vi "WristExecuteLogic.vi"(8 "error in (no error)":errorcluster, 11 "EncoderPos (deg)":dbl) -> (0 "error out":errorcluster, 3 "MotorDmd":dbl)   [LabVIEW 2023]
uses:
  <vilib>/Rock Robotics/WPI/ThirdParty/JAS_Junk/TrajLib/VI/BoolCmd_Recv_Internal.vi
  <vilib>/Rock Robotics/WPI/ThirdParty/JAS_Junk/TrajLib/Util_GetTime.vi
  <vilib>/Rock Robotics/WPI/ThirdParty/JAS_Junk/TrajLib/VI/MathUtil_RateOfChange.vi
  <vilib>/Rock Robotics/WPI/ThirdParty/JAS_Junk/TrajLib/VI/BoolCmd_ObtainQueue.vi
  <vilib>/Rock Robotics/WPI/ThirdParty/JAS_Junk/TrajLib/VI/Util_GetTime_U32.vi
  Elevator/ElevatorGlobal.vi
  WristGlobal.vi
  <vilib>/Rock Robotics/SystemInterfaces/Utilities/FPGA_UtilitiesRead LocalTime.vi
  <vilib>/Rock Robotics/WPI/ThirdParty/JAS_Junk/TrajLib/VI/Util_GetTime_U64.vi
  <vilib>/Rock Robotics/WPI/ThirdParty/JAS_Junk/TrajLib/Trajectory_Library.lvlib
  <vilib>/Rock Robotics/WPI/ThirdParty/JAS_Junk/TrajLib/Enum/DCMOTOR_TYPES_ENUM.ctl
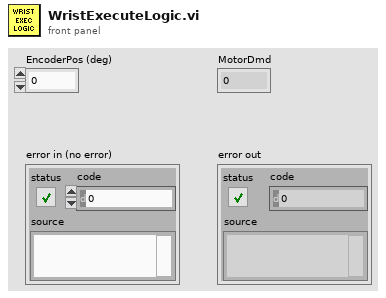
[diagram p1: front panel]
types:
  T1 = typedef "Trajectory_Library.lvlib/DCMOTOR_TYPES_ENUM.ctl" = enum16{"CIM", "AndyMark 9015", "Andy Mark RS 775 125", "Bag", "BaneBots RS 550", "BaneBots RS 775", "Falcon 500", "Mini CIM", "NEO", "NEO 550", "Romi BuiltIn", "Vex 775 Pro", "Snow Blower AM 2235A", "Bosch Seat AM 3493", "Falcon 500 FOC", "Kraken X60", "Kraken X60 FOC", "NEO Vortex"}
  T2 = typedef "Trajectory_Library.lvlib/LINEAR_SYSTEM_ID_SINGLE_JOINT_ARM_MODEL.ctl" = cluster{"DCMOTOR_TYPES":T1, "Num Motors":i32, "ArmLength_M":dbl, "massKg":dbl, "Gearing":dbl, "MOI kgm2":dbl, "Estimate MOI":bool}
  T3 = typedef "Trajectory_Library.lvlib/LINEAR_SYSTEM_LOOP_SNGJNTARM_CTRL_PARAMS.ctl" = cluster{"Ang Model Std Dev Rad":dbl, "Ang Meas Std Dev Rad":dbl, "Ang Ctrl Tol Rad":dbl, "Max Ctrl Out V":dbl, "Vel Model Std Dev Rad/Sec":dbl, "Vel Ctrl Tol Rad/Sec":dbl}
  T4 = typedef "Trajectory_Library.lvlib/PosCtrl_Tuning_Type.ctl" = cluster{"Slope":dbl, "Offset":dbl, "Error Deadband":dbl, "At Reference Count":i32, "Negate Output":bool, "Max Allowd Position":dbl, "Min Allowd Position":dbl, "Kd":dbl, "FilterDerivative":bool}
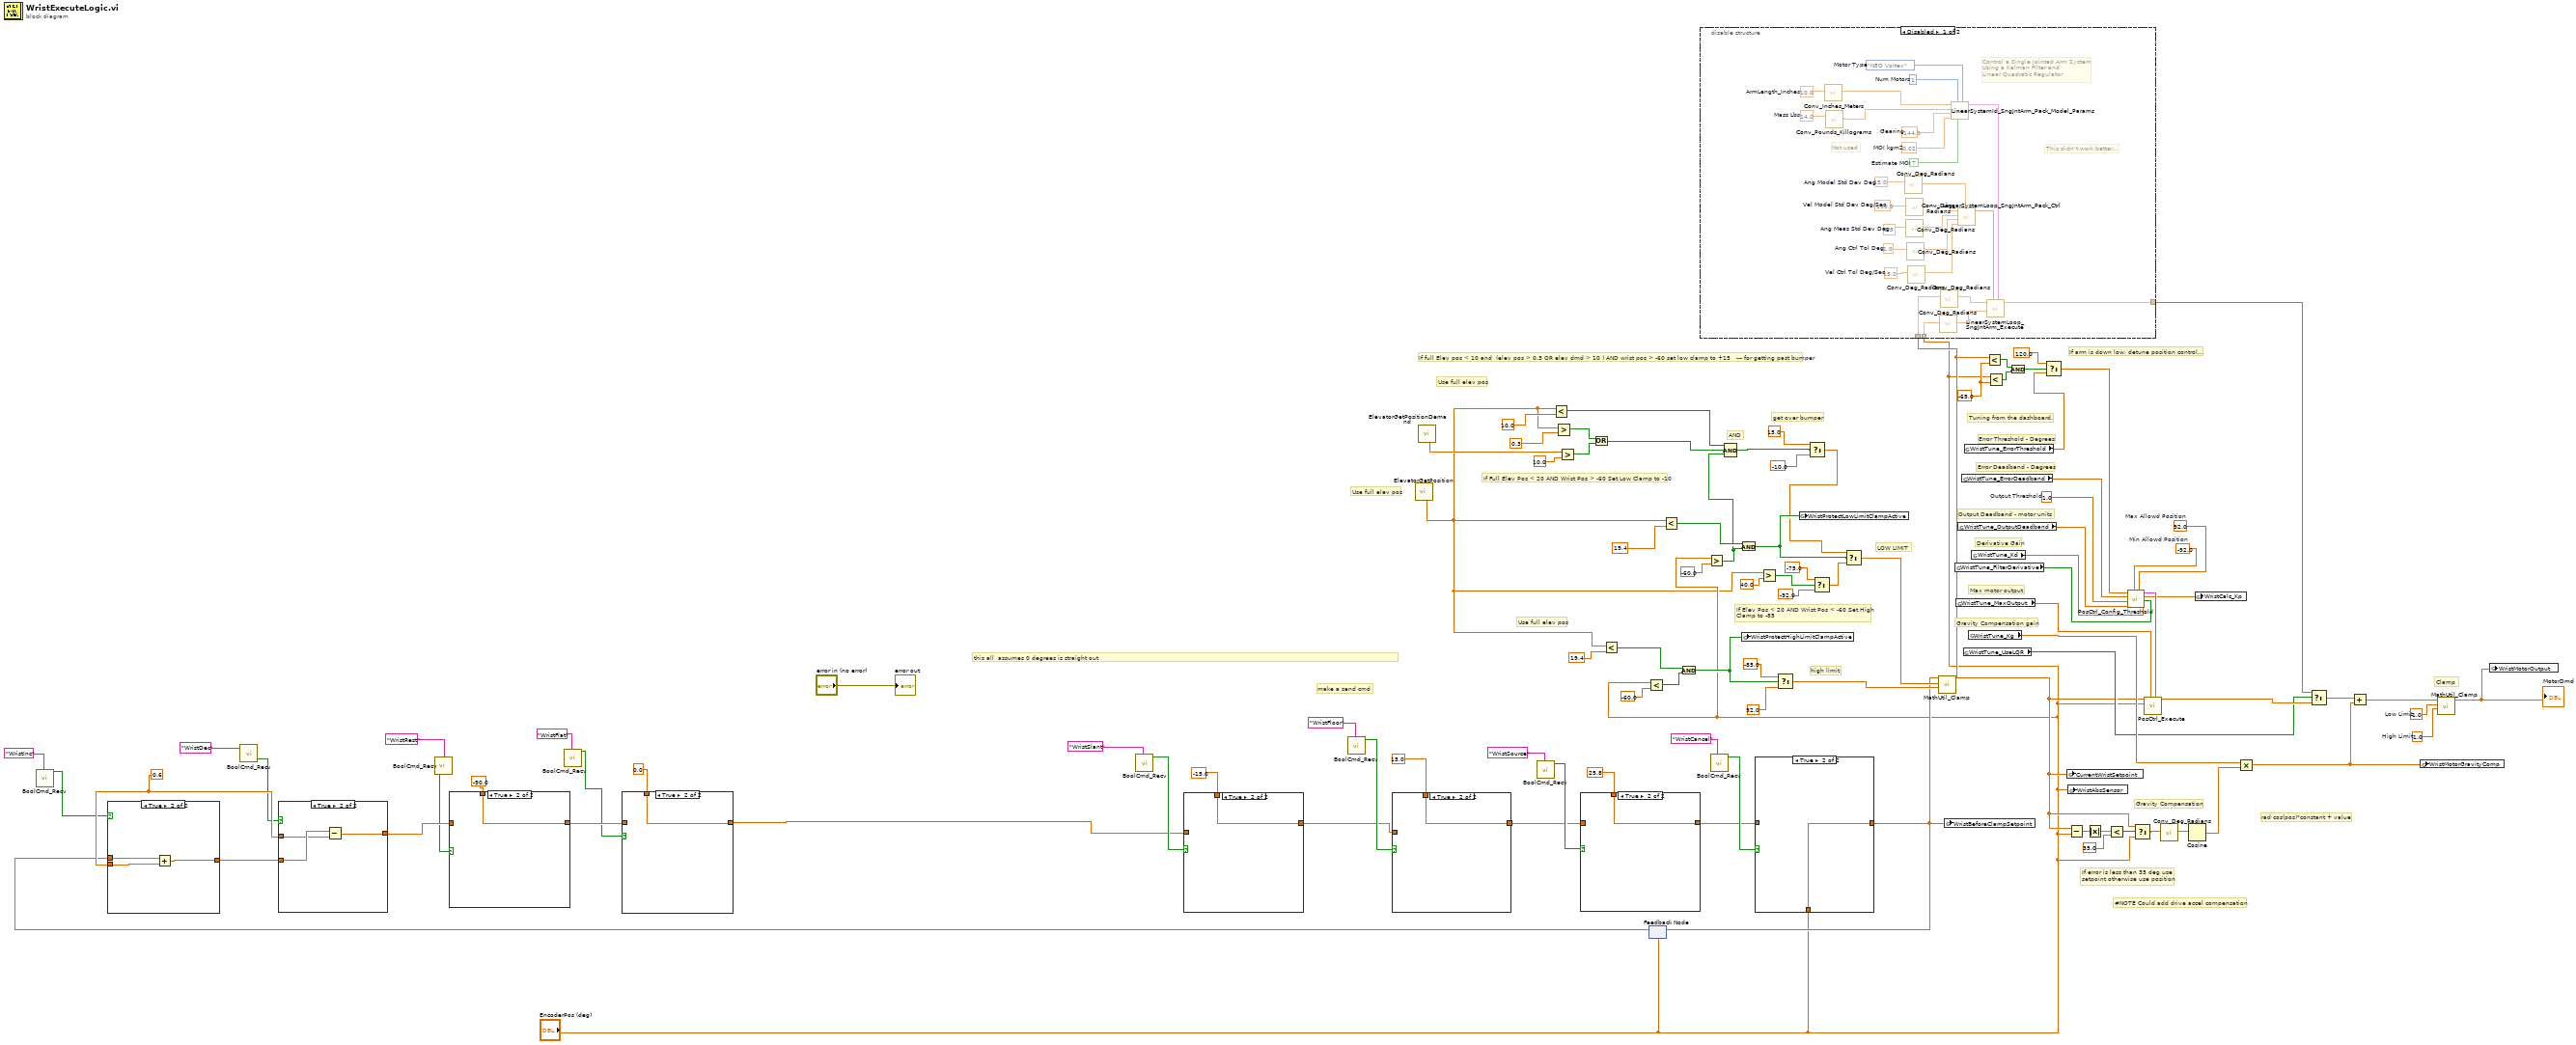
[diagram p0: block diagram]
diagram:
  w26 = -92.0  # Min Allowd Position
  w27 = 92.0  # Max Allowd Position
  w36 = -65.0 ("y")
  w99 = 1.0  # Output Threshold
  w97 = 1.0  # High Limit
  w98 = -1.0  # Low Limit
  w93 = 0.6 ("x")
  # "make a send cmd"
  # "LOW LIMIT"
  # "get over bumper"
  # "AND"
  # "Use full elev pos"
  # "If full Elev pos < 10 and  (elev pos > 0.3 OR elev dmd > 10 ) AND wrist pos > -60 set low clamp to +15   --- for getting past bumper"
  # "#NOTE Could add drive accel compensation"
  # "Use full elev pos"
  # "Use full elev pos"
  # "If arm is down low, detune position control..."
  # "If error is less than 35 deg use\nsetpoint otherwise use position"
  # "Gravity Compensation gain"
  # "Tuning from the dashboard."
  # "Max motor output"
  # "Derivative Gain"
  # "Output Deadband - motor units"
  # "Error Deadband - Degrees"
  # "Error Threshold - Degrees"
  # "If Elev Pos < 20 AND Wrist Pos < -60 Set High\nClamp to -85"
  # "If Full Elev Pos < 20 AND Wrist Pos > -60 Set Low Clamp to -10"
  # "high limit"
  # "Gravity Compensation"
  # "rad cos(pos)*constant + value"
  # "Clamp"
  # "this all  assumes 0 degrees is straight out"
  n1 = call <vilib>:"BoolCmd_Recv.vi"("Command Name"="WristInc") -> ("New Request"=w82:bool)  [unwired: 9 in, 1 out]
  n2 = call <vilib>:"BoolCmd_Recv.vi"("Command Name"="WristDec") -> ("New Request"=w84:bool)  [unwired: 9 in, 1 out]
  n3 = call <vilib>:"BoolCmd_Recv.vi"("Command Name"="WristRest") -> ("New Request"=w80:bool)  [unwired: 9 in, 1 out]
  n4 = call <vilib>:"BoolCmd_Recv.vi"("Command Name"="WristFlat") -> ("New Request"=w86:bool)  [unwired: 9 in, 1 out]
  n5 = call <vilib>:"BoolCmd_Recv.vi"("Command Name"="WristSlant") -> ("New Request"=w88:bool)  [unwired: 9 in, 1 out]
  n6 = call <vilib>:"BoolCmd_Recv.vi"("Command Name"="WristFloor") -> ("New Request"=w5:bool)  [unwired: 9 in, 1 out]
  n7 = call "ElevatorGetPosition.vi"() -> ("ElevFullHeight"=w10:dbl)  [unwired: 9 in, 2 out]
  n8 = call "ElevatorGetPositionDemand.vi"() -> ("ElevatorFullDmdInches"=w17:dbl)  [unwired: 8 in, 2 out]
  n9 = call <vilib>:"BoolCmd_Recv.vi"("Command Name"="WristSource") -> ("New Request"=w59:bool)  [unwired: 9 in, 1 out]
  n10 = Less?(x=w10, y=10.0) -> (x < y?=w23:bool)
  n11 = Greater?(x=w10, y=0.3) -> (0:w15:bool)
  n12 = Greater?(x=w17, y=10.0) -> (0:w14:bool)
  n13 = Or(x=w15, y=w14) -> (x .or. y?=w13:bool)
  n14 = Less?(x=w10, y=19.4) -> (x < y?=w67:bool)
  n15 = Less?(x="EncoderPos (deg)", y=-60.0) -> (x < y?=w65:bool)
  n16 = feedback #1("EncoderPos (deg)") -> (w89:dbl)
  n17 = case shown="True" w82 {
    tunnel: w89 -> [w101 w103]
    tunnel: [w101 w104] -> w90
    tunnel: w93 -> [_ w102]
    frame False {
    }
    frame True {
      n18 = Add(x=w103, y=w102) -> (x+y=w104:dbl)
    }
  }
  n19 = case shown="True" w84 {
    tunnel: w90 -> [w105 w107]
    tunnel: [w105 w108] -> w91
    tunnel: w93 -> [_ w106]
    frame False {
    }
    frame True {
      n20 = Subtract(x=w107, y=w106) -> (x-y=w108:dbl)
    }
  }
  n21 = case shown="True" w80 {
    tunnel: w91 -> [w109 _]
    tunnel: [w109 w110] -> w92
    tunnel: -90.0 ("Numeric") -> [_ w110]
    frame False {
    }
    frame True {
    }
  }
  n22 = case shown="True" w86 {
    tunnel: w92 -> [w111 _]
    tunnel: [w111 w112] -> w1
    tunnel: 0.0 ("Result") -> [_ w112]
    frame False {
    }
    frame True {
    }
  }
  n23 = case shown="True" w88 {
    tunnel: w1 -> [w113 _]
    tunnel: [w113 w114] -> w4
    tunnel: -15.0 ("Result") -> [_ w114]
    frame False {
    }
    frame True {
    }
  }
  n24 = case shown="True" w5 {
    tunnel: w4 -> [w115 _]
    tunnel: [w115 w116] -> w3
    tunnel: 15.0 ("Result") -> [_ w116]
    frame False {
    }
    frame True {
    }
  }
  n25 = case shown="True" w59 {
    tunnel: [w117 w118] -> w57
    tunnel: 25.8 ("Result") -> [_ w118]
    tunnel: w3 -> [w117 _]
    frame False {
    }
    frame True {
    }
  }
  n26 = Less?(x=w10, y=19.4) -> (x < y?=w63:bool)
  n27 = And(x=w67, y=w65) -> (x .and. y?=w54:bool)
  n28 = Greater?(x="EncoderPos (deg)", y=-60.0) -> (0:w22:bool)
  n29 = call <vilib>:"BoolCmd_Recv.vi"("Command Name"="WristCancel") -> ("New Request"=w77:bool)  [unwired: 9 in, 1 out]
  n30 = Compound Arithmetic op=AND(w23, w13, w22) -> (w19:bool)
  n31 = And(x=w63, y=w22) -> (x .and. y?=w55:bool)
  n32 = global write "WristGlobal.vi" "WristProtectHighLimitClampActive"(w54) -> ()
  n33 = case shown="True" w77 {
    tunnel: w57 -> [w119 _]
    tunnel: [w119 w120] -> w56
    tunnel: "EncoderPos (deg)" -> [_ w120]
    frame False {
    }
    frame True {
    }
  }
  n34 = feedback-in #1(w56) -> ()
  n35 = Greater?(x=w10, y=40.0) -> (0:w8:bool)
  n36 = Select(t=-85.0, s=w54, f=92.0) -> (s? t:f=w68:dbl)
  n37 = global write "WristGlobal.vi" "WristProtectLowLimitClampActive"(w55) -> ()
  n38 = Select(t=15.0, s=w19, f=-10.0 ("t")) -> (s? t:f=w18:dbl)
  n39 = Select(t=-75.0, s=w8, f=-92.0) -> (s? t:f=w11:dbl)
  n40 = Select(t=w18, s=w55, f=w11) -> (s? t:f=w61:dbl)
  n41 = call <vilib>:"MathUtil_Clamp.vi"("High Limit"=w68, "Low Limit"=w61, "Value"=w56) -> ("Result"=w33:dbl)  [unwired: 8 in]
  n42 = disable-structure shown="Disabled" {
    disable-tunnel: [w123 _] -> w38
    disable-tunnel: w33 -> [w122 _]
    disable-tunnel: "EncoderPos (deg)" -> [w121 _]
    frame Disabled {
      w130 = 100.0  # Vel Model Std Dev Deg/Sec
      w129 = 0.5  # Ang Meas Std Dev Deg
      w128 = 1.0  # Ang Ctrl Tol Deg
      w127 = 15.0  # Vel Ctrl Tol Deg/Sec
      w132 = 25.0  # Ang Model Std Dev Deg
      w142 = TRUE  # Estimate MOI
      w143 = 0.02  # MOI kgm2
      w137 = 10.0  # ArmLength_Inches
      w144 = 144.0  # Gearing
      w135 = 14.0  # Mass Lbs
      w145 = 1  # Num Motors
      w146 = DCMOTOR_TYPES_ENUM."NEO Vortex"  # Motor Type
      # "This didn't work better..."
      # "Not used"
      # "Control a Single Jointed Arm System\nUsing a Kalman Filter and \nLinear Quadratic Regulator"
      n43 = call <vilib>:"Conv_Inches_Meters.vi"("INCH"=w137) -> ("Meters"=w136:dbl)  [unwired: 10 in]
      n44 = call <vilib>:"Conv_Pounds_Killograms.vi"("Pounds"=w135) -> ("Killograms"=w134:dbl)  [unwired: 10 in]
      n45 = call <vilib>:"Conv_Deg_Radians.vi"("Degress"=w132) -> ("Radians"=w133:dbl)  [unwired: 10 in]
      n46 = call <vilib>:"Conv_Deg_Radians.vi"("Degress"=w129) -> ("Radians"=w126:dbl)  [unwired: 10 in]
      n47 = call <vilib>:"Conv_Deg_Radians.vi"("Degress"=w130) -> ("Radians"=w131:dbl)  [unwired: 10 in]
      n48 = call <vilib>:"Conv_Deg_Radians.vi"("Degress"=w128) -> ("Radians"=w125:dbl)  [unwired: 10 in]
      n49 = call <vilib>:"Conv_Deg_Radians.vi"("Degress"=w127) -> ("Radians"=w124:dbl)  [unwired: 10 in]
      n50 = call <vilib>:"Conv_Deg_Radians.vi"("Degress"=w121) -> ("Radians"=w139:dbl)  [unwired: 10 in]
      n51 = call <vilib>:"Conv_Deg_Radians.vi"("Degress"=w122) -> ("Radians"=w138:dbl)  [unwired: 10 in]
      n52 = call <vilib>:"LinearSystemId_SngJntArm_Pack_Model_Params.vi"("DCMOTOR_TYPES"=w146, "Estimate MOI"=w142, "Num Motors"=w145, "MOI kgm2"=w143, "Gearing"=w144, "massKg"=w134, "ArmLength_M"=w136) -> ("SngJntArmSim_Model _Params"=w141:T2)  [unwired: 4 in]
      n53 = call <vilib>:"LinearSystemLoop_SngJntArm_Pack_Ctrl.vi"("Ang Model Std Dev Rad"=w133, "Vel Ctrl Tol Rad/Sec"=w124, "Ang Ctrl Tol Rad"=w125, "Ang Meas Std Dev Rad"=w126, "Vel Model Std Dev Rad/Sec"=w131) -> ("LinearSystemLoop_SngJntArm_Ctrl_Params"=w140:T3)  [unwired: 6 in]
      n54 = call <vilib>:"LinearSystemLoop_SngJntArm_Execute.vi"("LinearSystem_ID_SngJntArm_Model"=w141, "LinearSystem_SngJntArm_Ctrl_Params"=w140, "Process Variable\nRadians"=w139, "Ang Pos SP Rad"=w138) -> ("Motor Dmd"=w123:dbl)  [unwired: 3 in, 4 out]
    }
    frame Enabled {
    }
  }
  n55 = global write "WristGlobal.vi" "WristBeforeClampSetpoint"(w56) -> ()
  n56 = global read "WristGlobal.vi" "WristTune_FilterDerivative"() -> (w48:bool)
  n57 = global read "WristGlobal.vi" "WristTune_MaxOutput"() -> (w50:dbl)
  n58 = global read "WristGlobal.vi" "WristTune_OutputDeadband"() -> (w52:dbl)
  n59 = global read "WristGlobal.vi" "WristTune_ErrorDeadband"() -> (w53:dbl)
  n60 = global read "WristGlobal.vi" "WristTune_UseLQR"() -> (w37:bool)
  n61 = global read "WristGlobal.vi" "WristTune_ErrorThreshold"() -> (w28:dbl)
  n62 = global read "WristGlobal.vi" "WristTune_Kg"() -> (w43:dbl)
  n63 = global read "WristGlobal.vi" "WristTune_Kd"() -> (w51:dbl)
  n64 = Less?(x=w33, y=w36) -> (x < y?=w34:bool)
  n65 = Less?(x="EncoderPos (deg)", y=w36) -> (x < y?=w35:bool)
  n66 = And(x=w34, y=w35) -> (x .and. y?=w31:bool)
  n67 = Select(t=120.0, s=w31, f=w28) -> (s? t:f=w30:dbl)
  n68 = global write "WristGlobal.vi" "CurrentWristSetpoint"(w33) -> ()
  n69 = global write "WristGlobal.vi" "WristAbsSensor"("EncoderPos (deg)") -> ()
  n70 = Subtract(x=w33, y="EncoderPos (deg)") -> (x-y=w47:dbl)
  n71 = Absolute Value(x=w47) -> (abs(x)=w46:dbl)
  n72 = Less?(x=w46, y=35.0) -> (x < y?=w44:bool)
  n73 = call <vilib>:"PosCtrl_Config_Threshold.vi"("Kd"=w51, "FilterDerivative"=w48, "Max Allowd Position"=w27, "Min Allowd Position"=w26, "Output Deadband"=w52, "Output Threshold"=w99, "ErrorDeadband"=w53, "ErrorThreshold"=w30) -> ("Kp"=w49:dbl, "PosCtrl_Config_Params"=w96:T4)  [unwired: 2 in]
  n74 = Select(t=w33, s=w44, f="EncoderPos (deg)") -> (s? t:f=w42:dbl)
  n75 = call <vilib>:"PosCtrl_Execute.vi"("PosCtrl_Config_Params"=w96, "MaxOutput"=w50, "CurrentPosition"="EncoderPos (deg)", "TargetPosition"=w33) -> ("Output"=w40:dbl)  [unwired: 5 in, 2 out]
  n76 = call <vilib>:"Conv_Deg_Radians.vi"("Degress"=w42) -> ("Radians"=w72:dbl)  [unwired: 10 in]
  n77 = Cosine(x=w72) -> (cos(x)=w41:dbl)
  n78 = global write "WristGlobal.vi" "WristCalc_Kp"(w49) -> ()
  n79 = Multiply(x=w43, y=w41) -> (x*y=w69:dbl)
  n80 = Select(t=w38, s=w37, f=w40) -> (s? t:f=w39:dbl)
  n81 = Add(x=w39, y=w69) -> (x+y=w71:dbl)
  n82 = global write "WristGlobal.vi" "WristMotorGravityComp"(w69) -> ()
  n83 = call <vilib>:"MathUtil_Clamp.vi"("High Limit"=w97, "Low Limit"=w98, "Value"=w71) -> ("Result"=w70:dbl)  [unwired: 8 in]
  "MotorDmd" <- w70
  n84 = global write "WristGlobal.vi" "WristMotorOutput"(w70) -> ()
  "error out" <- "error in (no error)"
